vi "Example4_Week2.vi"() -> ()   [LabVIEW 2015]
panel:
  out "Numeric":dbl
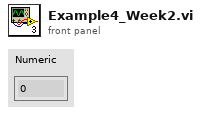
[diagram p1: front panel]
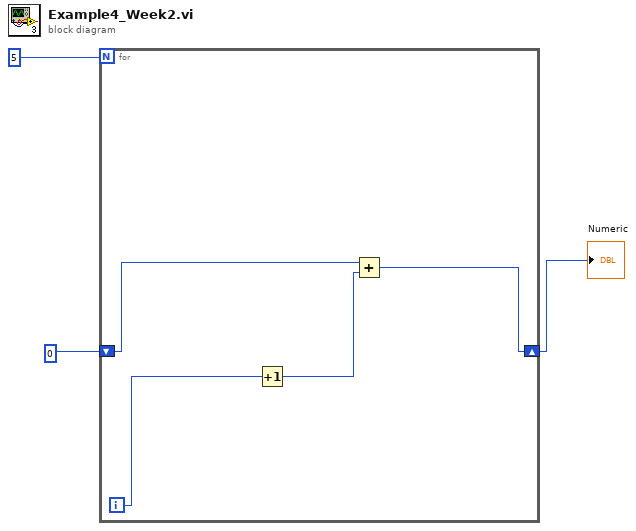
[diagram p0: block diagram]
diagram:
  n1 = for {
    N: 5 -> [_]
    shift-right: [w4] -> w1
    shift-left: 0 -> [w5]
    i -> [w7]
    n2 = Increment(x=w7) -> (x+1=w6:i32)
    n3 = Add(x=w5, y=w6) -> (x+y=w4:i32)
  }
  "Numeric" <- w1
